vi "Initialize.vi"(11 "Port Number":i16=1 min=0 max=20) -> (0 "error out":errorcluster, 1 "Instrument Info":string[](array[string]), 2 "OK ?":bool, 3 "Visa Session":refnum<visa-resource-name>, 4 "Range Info":T1, 5 "Units":string)   [LabVIEW 2020, in "Ophir Power Meter.lvlib"]
uses:
  Ophir Power Meter.lvlib
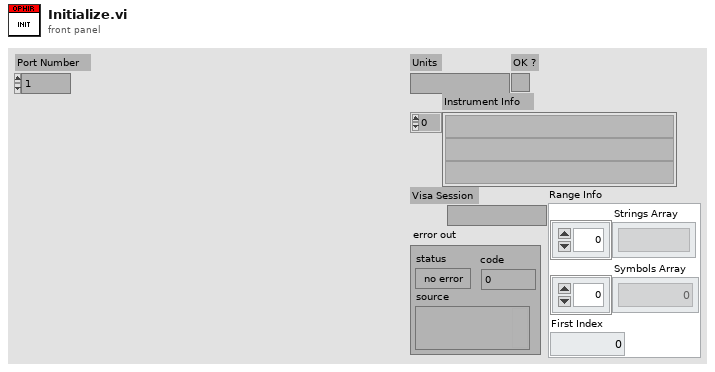
[diagram p1: front panel]
types:
  T1 = cluster{"Strings Array":string[], "Symbols Array":i32[], "First Index":i32}
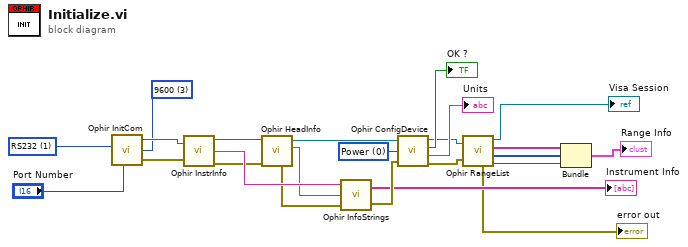
[diagram p0: block diagram]
diagram:
  w9 = i16 3 items=["300", "1200", "4800", "9600", "19200", "38400"] ("Baud Rate (3:9600)")
  w13 = u16 0 items=["Power", "Energy", "Frequency"] ("Measure Choice (0:Power)")
  w24 = i16 1 items=["USB", "RS232", "GPIB"] ("Communication (default USB 0)")
  n1 = call <instrlib>:"Ophir InitCom.vi"("Communication (default USB 0)"=w24, "Port Number (default 2)"="Port Number", "Baud Rate (3:9600)"=w9) -> ("dup Visa Session"=w21:refnum<visa-resource-name>, "error out"=w22:errorcluster)  [unwired: 3 in, 1 out]
  n2 = call <instrlib>:"Ophir InstrInfo.vi"("Visa Session"=w21, "error in (no error)"=w22) -> ("dup Visa Session"=w18:refnum<visa-resource-name>, "Instrument Info"=w20:string, "error out"=w19:errorcluster)
  n3 = call <instrlib>:"Ophir HeadInfo.vi"("Visa Session"=w18, "error in (no error)"=w19) -> ("error out"=w16:errorcluster, "dup Visa Session"=w14:refnum<visa-resource-name>, "Head Info"=w17:string)  [unwired: 4 in, 2 out]
  n4 = call <instrlib>:"Ophir InfoStrings.vi"("error in (no error)"=w16, "Head Info"=w17, "Instrument Info"=w20) -> ("error out"=w15:errorcluster, "Strings Array"=→"Instrument Info":string[])
  n5 = call <instrlib>:"Ophir ConfigDevice.vi"("Visa Session"=w14, "Measure Choice (0:Power)"=w13, "error in (no error)"=w15) -> ("dup Visa Session"=w8:refnum<visa-resource-name>, "OK ?"=→"OK ?":bool, "Units"=→"Units":string, "error out"=w7:errorcluster)
  n6 = call <instrlib>:"Ophir RangeList.vi"("Visa Session"=w8, "error in (no error)"=w7) -> ("error out"=→"error out":errorcluster, "dup Visa Session"=→"Visa Session":refnum<visa-resource-name>, "Strings Array"=w4:string[], "Symbols Array"=w3:i32[], "First Index"=w2:i32)  [unwired: 1 in]
  n7 = Bundle("Strings Array"=w4, "Symbols Array"=w3, "First Index"=w2) -> (→"Range Info":T1)  [unwired: 1 in]
